vi "holding.vi"() -> ()   [LabVIEW 2019]
panel:
  in  "Wait (second) 2":sgl
  in  "No  Steps":i16
  out "outputdc 2":dbl[](array[numeric]) format="%.2f"
  in  "GPIB address dc meter 2":string
  out "dup directory path":path
  in  "GPIB address dc meter":string
  in  "GPIB  address  lockin":string
  in  "GPIB address magnet":string
  in  "GPIB address Temp controller":string
  in  "Wait (second)":sgl
  in  "No of Temp Steps":i16
  in  "folder name to save files":string
  out "outputtemp":dbl[](array[numeric]) format="%.2f"
  out "outputdc":dbl[](array[numeric]) format="%.2f"
  out "outputlockin 2":dbl[](array[numeric]) format="%.2f"
  out "outputlockin 1":dbl[](array[numeric]) format="%.2f"
  out "field":dbl[](array[numeric]) format="%.2f"
  out "Current Temp":dbl format="%.3f"
  in  "Increasing \nTemp step":bool=TRUE
  in  "Temperature\nInterval":dbl format="%.3f"
  in  "Initial Temp C":dbl format="%.3f"
  # "Help:\n1. write the folder name to save the files.The file name will \nbe the temperature in the given folder.\n2.Write the GPIB address of all the instruments before running\nthe program.\n3. Give the initial temperature and the temperature interval \nand the total number of steps.\n4.Check whether you want to increase the temperature or\ndecrease.\n5.Write the time to be waited to let the tempetature controller\nequilibrate.\n6.Once the speps 1 through 5 is done run the experiment."
  # "Decreasing\nTemp Step"
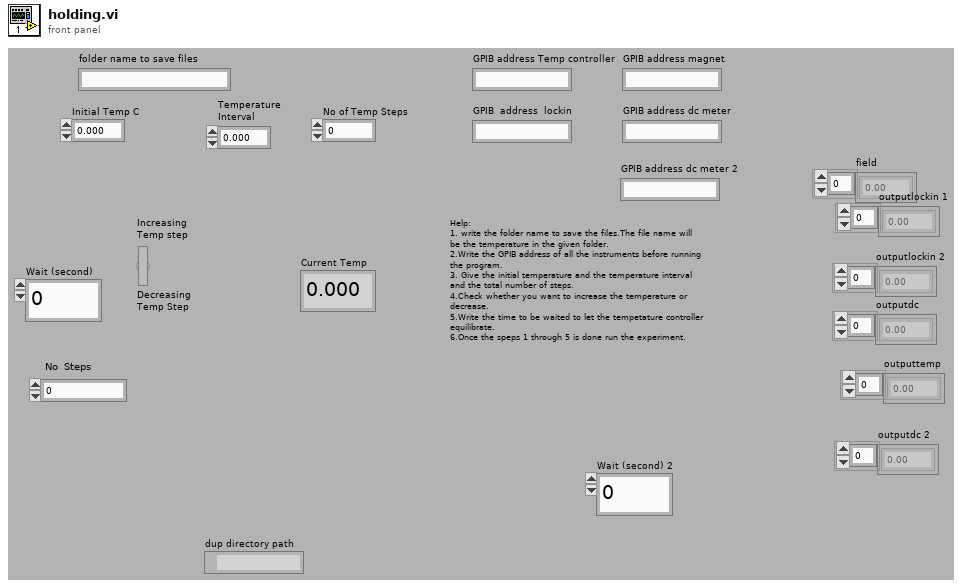
[diagram p1: front panel]
types:
  T1 = enum16{"--Quit--", "Read-Status", "Read-Cell", "Read-Field[T]", "Read-Setpoint[T]"}
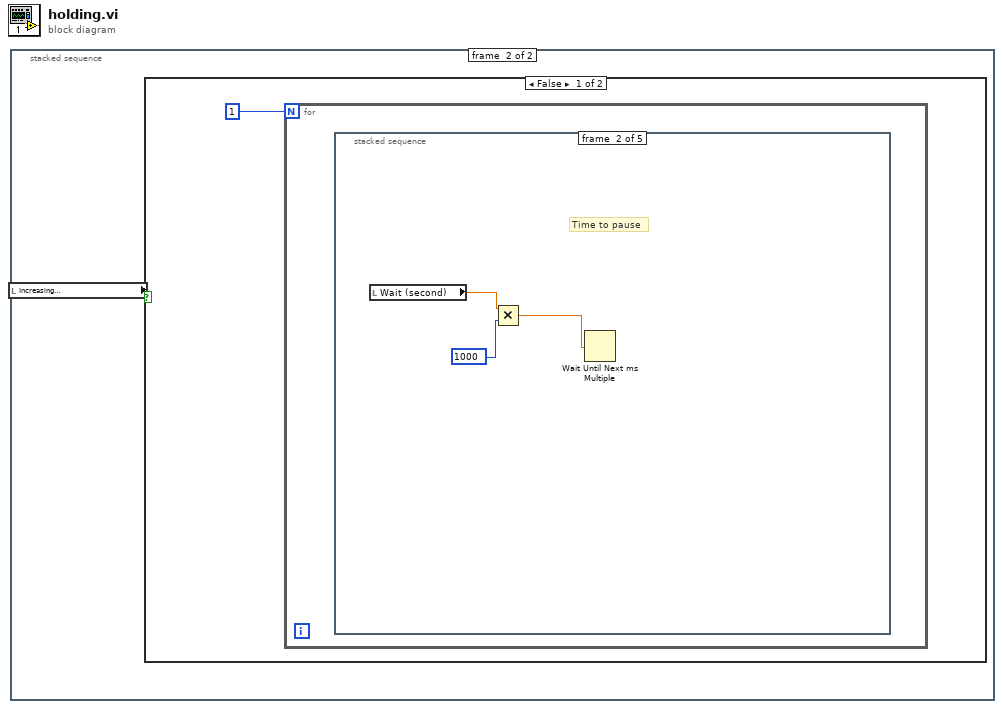
[diagram p0: block diagram]
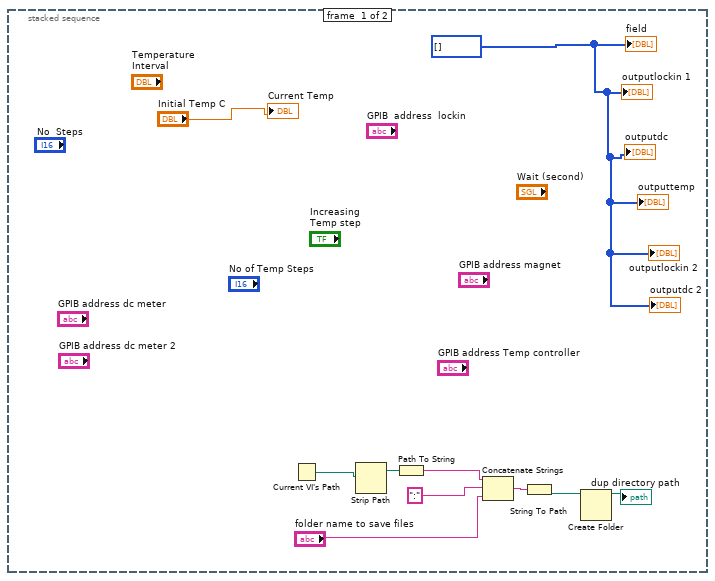
[diagram p2: hidden frame]
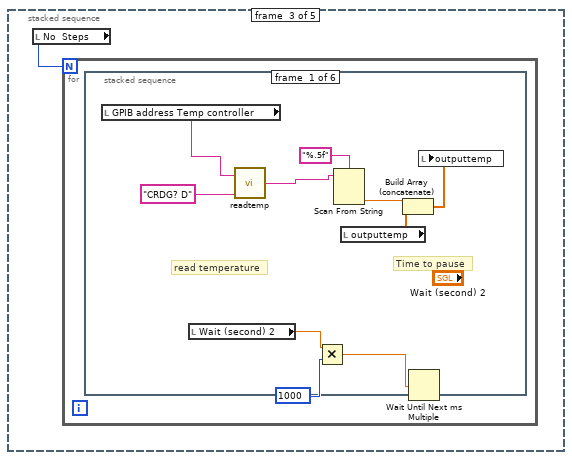
[diagram p4: hidden frame]
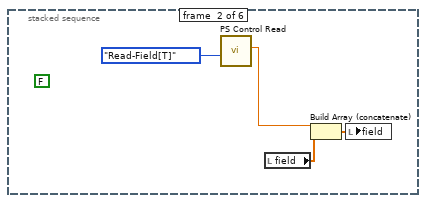
[diagram p5: hidden frame]
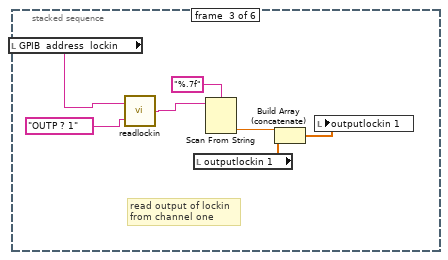
[diagram p6: hidden frame]
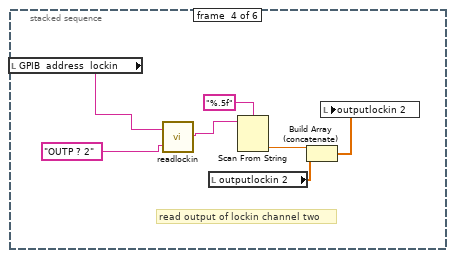
[diagram p7: hidden frame]
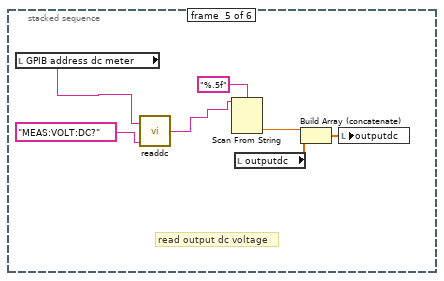
[diagram p8: hidden frame]
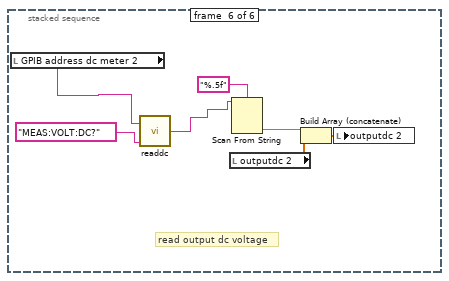
[diagram p9: hidden frame]
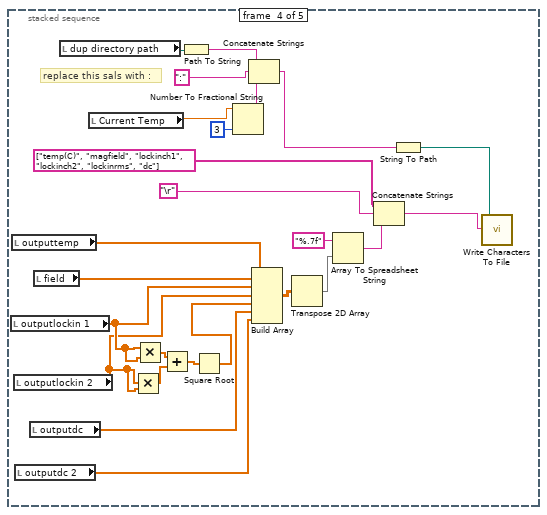
[diagram p10: hidden frame]
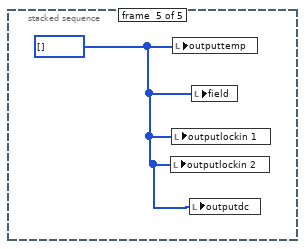
[diagram p11: hidden frame]
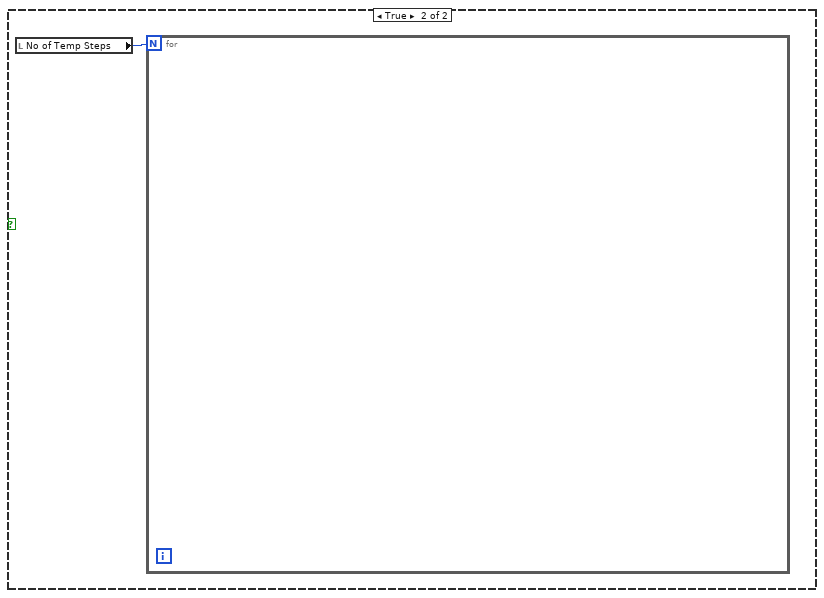
[diagram p12: hidden frame]
diagram:
  n1 = stacked-sequence {
    frame #0 {
      w1 = i32[] [] ("field")
      n2 = Current VI's Path() -> (path=w9:path)
      n3 = Strip Path(path=w9) -> (stripped path=w8:path)  [unwired: 1 out]
      n4 = Path To String(path=w8) -> (string=w7:string)
      n5 = Concatenate Strings(w7, ":", "folder name to save files") -> (w4:string)
      n6 = String To Path(string=w4) -> (path=w3:path)
      n7 = Create Folder(path (use dialog)=w3) -> (created path=→"dup directory path":path)  [unwired: 2 in, 2 out]
      "Current Temp" <- "Initial Temp C"
      "field" <- w1
      "outputlockin 1" <- w1
      "outputdc" <- w1
      "outputtemp" <- w1
      "outputlockin 2" <- w1
      "outputdc 2" <- w1
    }
    frame #1 {
      n8 = local read "Increasing \nTemp step"() -> (w11:bool)
      n9 = case shown="False" w11 {
        frame False {
          n10 = for {
            N: 1 -> [_]
            n11 = stacked-sequence {
              frame #0 {
              }
              frame #1 {
                # "Time to pause"
                n12 = local read "Wait (second)"() -> (w15:sgl)
                n13 = Multiply(x=w15, y=u32 1000 ("millisecond multiple")) -> (x*y=w13:sgl)
                n14 = Wait Until Next ms Multiple(millisecond multiple=w13) -> ()  [unwired: 1 out]
              }
              frame #2 {
                n15 = local read "No  Steps"() -> (w16:i16)
                n16 = for {
                  N: w16 -> [_]
                  n17 = stacked-sequence {
                    frame #0 {
                      # "Time to pause"
                      # "read temperature"
                      n18 = local read "GPIB address Temp controller"() -> (w20:string)
                      n19 = local read "Wait (second) 2"() -> (w19:sgl)
                      n20 = call "readtemp.vi"("Characters to Write"="CRDG? D", "GPIB\nAddress"=w20) -> ("Characters Read"=w21:string)
                      n21 = Multiply(x=w19, y=u32 1000 ("millisecond multiple")) -> (x*y=w17:sgl)
                      n22 = Scan From String(format string="%.5f", input string=w21) -> (output 1=w23:dbl)  [unwired: 3 in, 3 out]
                      n23 = local read "outputtemp"() -> (w26:dbl[])
                      n24 = Build Array (concatenate)(w23, w26) -> (w25:dbl[])
                      n25 = Wait Until Next ms Multiple(millisecond multiple=w17) -> ()  [unwired: 1 out]
                      n26 = local write "outputtemp"(w25) -> ()
                    }
                    frame #1 {
                      (unwired) FALSE
                      n27 = call "PS Control Read.vi"("Read State"=T1."Read-Field[T]") -> ("Current Field"=w27:dbl)  [unwired: 3 in, 4 out]
                      n28 = local read "field"() -> (w29:dbl[])
                      n29 = Build Array (concatenate)(w27, w29) -> (w28:dbl[])
                      n30 = local write "field"(w28) -> ()
                    }
                    frame #2 {
                      # "read output of lockin\nfrom channel one"
                      n31 = local read "GPIB  address  lockin"() -> (w31:string)
                      n32 = call "readlockin.vi"("Characters to Write"="OUTP ? 1", "GPIB\nAddress"=w31) -> ("Characters Read"=w32:string)
                      n33 = local read "outputlockin 1"() -> (w36:dbl[])
                      n34 = Scan From String(format string="%.7f", input string=w32) -> (output 1=w33:dbl)  [unwired: 3 in, 3 out]
                      n35 = Build Array (concatenate)(w33, w36) -> (w35:dbl[])
                      n36 = local write "outputlockin 1"(w35) -> ()
                    }
                    frame #3 {
                      # "read output of lockin channel two"
                      n37 = local read "GPIB  address  lockin"() -> (w38:string)
                      n38 = call "readlockin.vi"("Characters to Write"="OUTP ? 2", "GPIB\nAddress"=w38) -> ("Characters Read"=w39:string)
                      n39 = local read "outputlockin 2"() -> (w43:dbl[])
                      n40 = Scan From String(format string="%.5f", input string=w39) -> (output 1=w41:dbl)  [unwired: 3 in, 3 out]
                      n41 = Build Array (concatenate)(w41, w43) -> (w42:dbl[])
                      n42 = local write "outputlockin 2"(w42) -> ()
                    }
                    frame #4 {
                      # "read output dc voltage"
                      n43 = local read "GPIB address dc meter"() -> (w45:string)
                      n44 = call "readdc.vi"("Characters to Write"="MEAS:VOLT:DC?", "GPIB\nAddress"=w45) -> ("Characters Read"=w46:string)
                      n45 = Scan From String(format string="%.5f", input string=w46) -> (output 1=w48:dbl)  [unwired: 3 in, 3 out]
                      n46 = local read "outputdc"() -> (w51:dbl[])
                      n47 = Build Array (concatenate)(w48, w51) -> (w50:dbl[])
                      n48 = local write "outputdc"(w50) -> ()
                    }
                    frame #5 {
                      # "read output dc voltage"
                      n49 = local read "GPIB address dc meter 2"() -> (w52:string)
                      n50 = call "readdc.vi"("Characters to Write"="MEAS:VOLT:DC?", "GPIB\nAddress"=w52) -> ("Characters Read"=w53:string)
                      n51 = local read "outputdc 2"() -> (w58:dbl[])
                      n52 = Scan From String(format string="%.5f", input string=w53) -> (output 1=w55:dbl)  [unwired: 3 in, 3 out]
                      n53 = Build Array (concatenate)(w55, w58) -> (w57:dbl[])
                      n54 = local write "outputdc 2"(w57) -> ()
                    }
                  }
                }
              }
              frame #3 {
                # "replace this sals with :"
                n55 = local read "outputlockin 1"() -> (w76:dbl[])
                n56 = local read "outputtemp"() -> (w78:dbl[])
                n57 = local read "outputlockin 2"() -> (w75:dbl[])
                n58 = local read "outputdc 2"() -> (w59:dbl[])
                n59 = local read "outputdc"() -> (w70:dbl[])
                n60 = local read "field"() -> (w77:dbl[])
                n61 = local read "dup directory path"() -> (w61:path)
                n62 = local read "Current Temp"() -> (w80:dbl)
                n63 = Multiply(x=w75, y=w75) -> (x*y=w73:dbl[])
                n64 = Multiply(x=w76, y=w76) -> (x*y=w74:dbl[])
                n65 = Add(x=w74, y=w73) -> (x+y=w72:dbl[])
                n66 = Path To String(path=w61) -> (string=w60:string)
                n67 = Square Root(x=w72) -> (sqrt(x)=w71:dbl[])
                n68 = Number To Fractional String(number=w80, precision (6)=i16 3) -> (F-format string=w79:string)  [unwired: 2 in]
                n69 = Concatenate Strings(w60, ":", w79) -> (w82:string)
                n70 = Build Array(w78, w77, w76, w75, w71, w70, w59) -> (w69:dbl[][])
                n71 = Transpose 2D Array(2D array=w69) -> (transposed array=w67:dbl[][])
                n72 = Array To Spreadsheet String(array=w67, 3:"%.7f" ("format string")) -> (spreadsheet string=w64:string)  [unwired: 1 in]
                n73 = Concatenate Strings(string[] ["temp(C)", "magfield", "lockinch1", "lockinch2", "lockinrms", "dc"], "\r", w64) -> (w63:string)
                n74 = String To Path(string=w82) -> (path=w81:path)
                n75 = call <vilib>:"Write Characters To File.vi"("character string"=w63, "file path (dialog if empty)"=w81) -> ()  [unwired: 3 in, 1 out]
              }
              frame #4 {
                w84 = i32[] []
                n76 = local write "outputlockin 2"(w84) -> ()
                n77 = local write "outputlockin 1"(w84) -> ()
                n78 = local write "outputtemp"(w84) -> ()
                n79 = local write "outputdc"(w84) -> ()
                n80 = local write "field"(w84) -> ()
              }
            }
          }
        }
        frame True {
          n81 = local read "No of Temp Steps"() -> (w85:i16)
          n82 = for {
            N: w85 -> [_]
          }
        }
      }
    }
  }
